vi "4.6.2.vi"() -> ()   [LabVIEW 2017]
panel:
  in  "数值":dbl
  in  "数值 2":dbl
  out "x+y":dbl
  in  "停止":bool
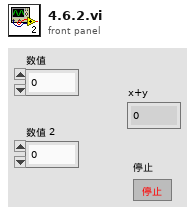
[diagram p1: front panel]
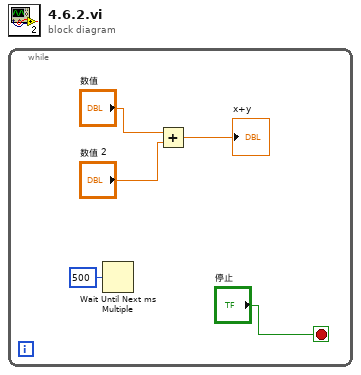
[diagram p0: block diagram]
diagram:
  n1 = while {
    stop <- "停止" stop-if-true
    n2 = Wait Until Next ms Multiple(millisecond multiple=500) -> ()  [unwired: 1 out]
    n3 = Add(x="数值", y="数值 2") -> (x+y=→"x+y":dbl)
  }
